vi "Init Events.vi"(8 "error in (no error)":errorcluster, 11 "Database in":refnum<class "Database.lvclass">) -> (0 "error out":errorcluster, 3 "Database out":refnum<class "Database.lvclass">)   [LabVIEW 2022 SP3, in "Database.lvclass"]
doc: "Developed by Kevin Thompson\nkevin@thompsonengineering.net\n\nCopyright 2018\nThompson Engineering, LLC"
uses:
  Database.lvclass
  Common/Controls/TD Async CmdMsg EventData--cluster.ctl
  Common/Controls/TD Sync API Event Data.ctl
  Common/Controls/APIReturnCluster--Cluster.ctl
  Common/Controls/TD Sync API Task State.ctl
  Database.lvclass/Database.ctl
  Accessors/Get PublicEvents.vi
  Accessors/Set PublicEvents.vi
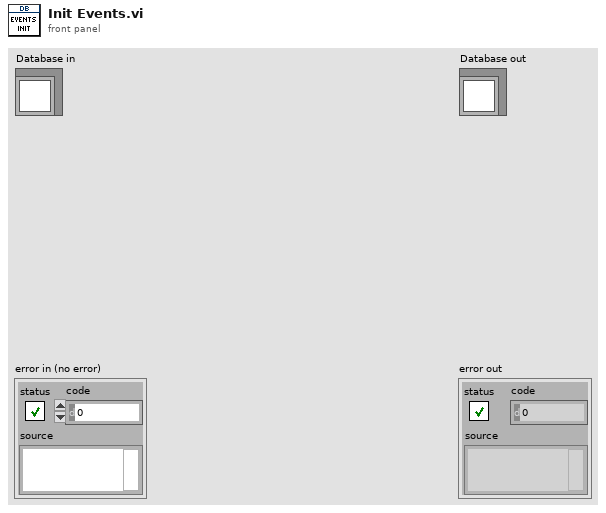
[diagram p1: front panel]
types:
  T1 = typedef "TD Sync API Event Data.ctl" = cluster{"Task":T2, "Command":variant, "Return Value":variant}
  T2 = typedef "APIReturnCluster--Cluster.ctl" = cluster{"Time Stamp":timestamp, "Timeout (ms)":u32, "Task State":T3, "Task Error":errorcluster, "Task ID":string, "Type":enum16{"API", "CMD"}}
  T3 = typedef "TD Sync API Task State.ctl" = enum16{"Completed", "Executing", "Errored", "Pending"}
  T4 = typedef "TD Async CmdMsg EventData--cluster.ctl" = cluster{"Time Stamp":timestamp, "CmdMsg":string, "vData":variant}
  T5 = typedef "Database.lvclass/Public Events--cluster.ctl" = cluster{"Temp01.AsyncCmd Event":refnum<user-event>, "Temp01.AsyncMsg Event":refnum<user-event>, "stop process":refnum<user-event>, "API Incoming Event":refnum<user-event>, "API Executed Event":refnum<user-event>, "API Return Event":refnum<user-event>}
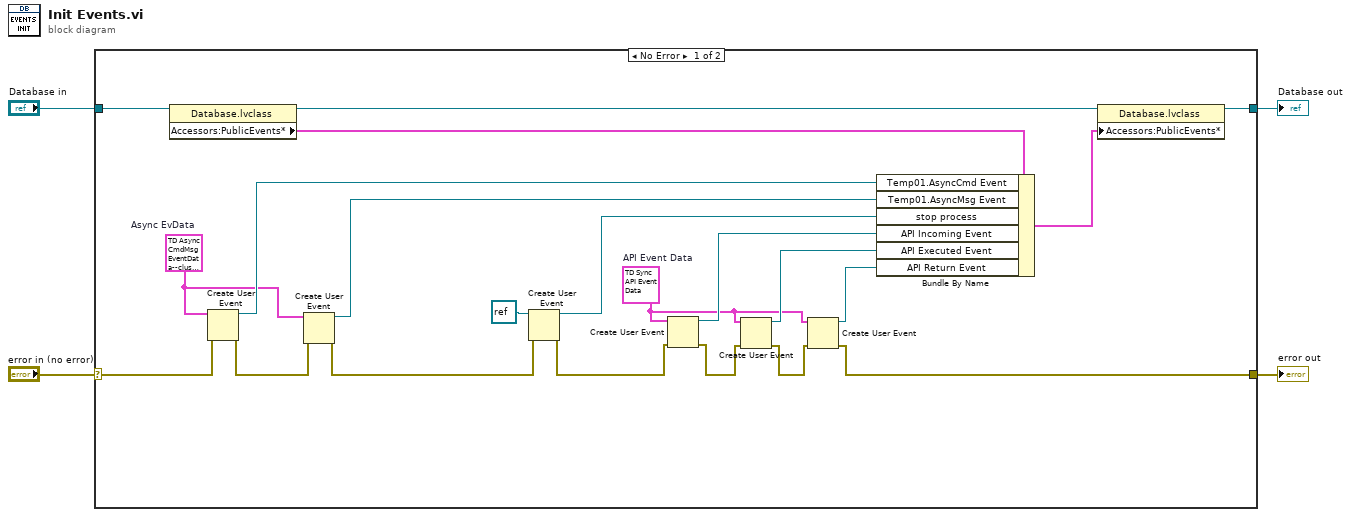
[diagram p0: block diagram]
diagram:
  n1 = case shown="No Error" "error in (no error)" {
    selector: "error in (no error)" -> [w18 w27]
    tunnel: [w6 w27] -> w3
    tunnel: [w25 w26] -> w1
    tunnel: "Database in" -> [w24 w26]
    frame No Error {
      w10 = T1 {"Task"={"Time Stamp"=timestamp(0 s since 1904-01-01), "Timeout (ms)"=0, "Task State"=enum."Completed", "Task Error"={"status"=FALSE, "code"=0, "source"=""}, "Task ID"="", "Type"=enum."API"}, "Command"=variant, "Return Value"=variant}  # API Event Data
      w15 = T4 {"Time Stamp"=timestamp(0 s since 1904-01-01), "CmdMsg"="", "vData"=variant}  # Async EvData
      n2 = property class="Database.lvclass"(reference=w24) -> (reference out=w23:refnum<class "Database.lvclass">, "Accessors:PublicEvents*"=w22:T5)  [unwired: 1 in, 1 out]
      n3 = Create User Event(user event datatype=w15, error in=w18) -> (user event=w19:refnum<user-event>, error out=w17:errorcluster)
      n4 = Create User Event(user event datatype=w15, error in=w17) -> (user event=w14:refnum<user-event>, error out=w16:errorcluster)
      n5 = Create User Event(user event datatype=refnum<notifier> refnum ("notifier out"), error in=w16) -> (user event=w20:refnum<user-event>, error out=w13:errorcluster)
      n6 = Create User Event(user event datatype=w10, error in=w13) -> (user event=w12:refnum<user-event>, error out=w8:errorcluster)
      n7 = Create User Event(user event datatype=w10, error in=w8) -> (user event=w11:refnum<user-event>, error out=w7:errorcluster)
      n8 = Create User Event(user event datatype=w10, error in=w7) -> (user event=w9:refnum<user-event>, error out=w6:errorcluster)
      n9 = Bundle By Name(cluster=w22, "Temp01.AsyncCmd Event"=w19, "Temp01.AsyncMsg Event"=w14, "stop process"=w20, "API Incoming Event"=w12, "API Executed Event"=w11, "API Return Event"=w9) -> (w5:T5)
      n10 = property class="Database.lvclass"(reference=w23, "Accessors:PublicEvents*"=w5) -> (reference out=w25:refnum<class "Database.lvclass">)  [unwired: 1 in, 1 out]
    }
    frame Error {
    }
  }
  "error out" <- w3
  "Database out" <- w1
